vi "Start.vi"(5 "ShowPanel?":bool, 6 "BcQueName":string, 7 "BusIndex":u32, 8 "error in (no error)":errorcluster, 9 "Script":string[](array[string]), 10 "Name":string, 11 "VI Refnum":refnum<vi>) -> (0 "error out":errorcluster, 2 "BC ID":i32, 3 "BCAdmin":refnum<class "BCAdmin.lvclass">)   [LabVIEW 2014, in "BusController.lvlib"]
uses:
  BusController.lvlib
  Admin/BCAdmin.lvclass
  Admin/BCAdmin.lvclass/BCAdmin.ctl
  Admin/Accessors/Write BC ID.vi
  Admin/Accessors/Write BCRegRef.vi
  Admin/Accessors/Write Name.vi
  Admin/Accessors/Write Script.vi
  Admin/Accessors/Write BusIndex.vi
  Admin/Accessors/Write BcQueName.vi
  Admin/Accessors/Write ShowPanel_.vi
  <vilib>/Utility/error.llb/Error Cluster From Error Code.vi
  <vilib>/ErrorRing/Error Ring.xnode
  Admin/Registry/BCReg.lvclass
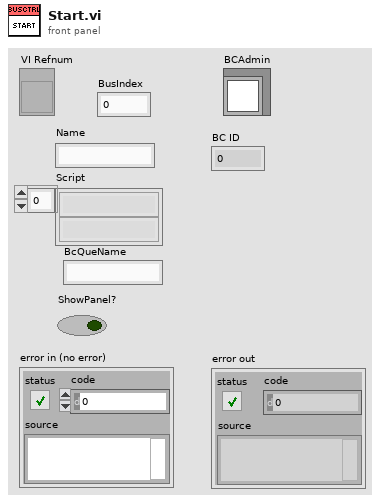
[diagram p1: front panel]
types:
  T1 = enum32{"Bad", "Idle", "Run top level", "Running"}
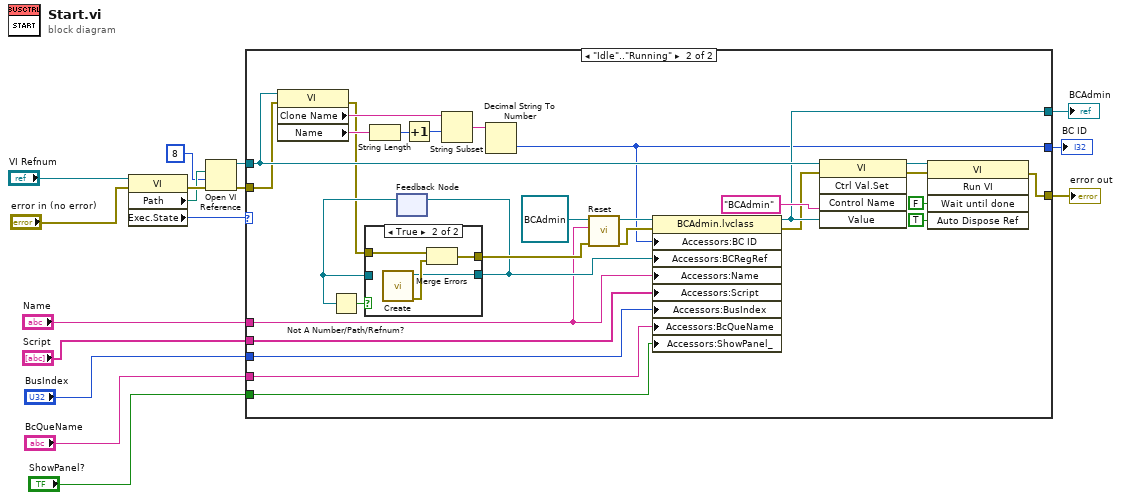
[diagram p0: block diagram]
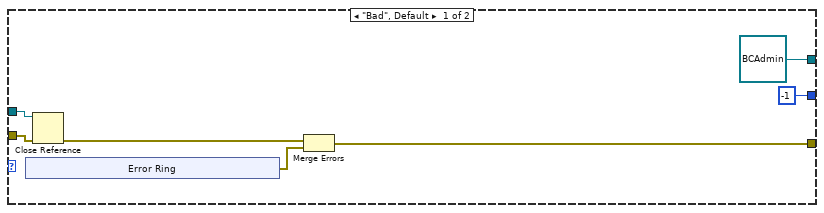
[diagram p2: hidden frame]
diagram:
  n1 = property class="VI"(reference="VI Refnum", error in="error in (no error)") -> (error out=w13:errorcluster, "Path"=w12:path, "Exec.State"=w14:T1)  [unwired: 1 out]
  n2 = Open VI Reference(vi path=w12, options=8, error in (no error)=w13) -> (vi reference=w9:refnum<vi>, error out=w10:errorcluster)  [unwired: 3 in]
  n3 = case shown="\"Idle\"..\"Running\"" w14 {
    tunnel: w10 -> [w22 w33]
    tunnel: w9 -> [w23 w43]
    tunnel: [w19 w37] -> w8
    tunnel: [refnum<class "BCAdmin.lvclass"> refnum ("BCAdmin") w36] -> w7
    tunnel: "Name" -> [_ w44]
    tunnel: [-1 w35] -> w5
    tunnel: "Script" -> [_ w34]
    tunnel: "BusIndex" -> [_ w30]
    tunnel: "BcQueName" -> [_ w29]
    tunnel: "ShowPanel?" -> [_ w28]
    frame "Bad", Default {
      n4 = xnode "Error Ring"() -> ("error out"=w20:errorcluster)
      n5 = Close Reference(reference=w23, error in (no error)=w22) -> (error out=w21:errorcluster)
      n6 = Merge Errors(w21, w20) -> (w19:errorcluster)
    }
    frame "Idle".."Running" {
      n7 = property class="VI"(reference=w43, error in=w33) -> (error out=w32:errorcluster, "Clone Name"=w55:string, "Name"=w52:string)  [unwired: 1 out]
      n8 = String Length(string=w52) -> (length=w53:i32)
      n9 = feedback #1() -> (w50:refnum<data-value>)  [unwired: 1 in]
      n10 = Not A Number/Path/Refnum?(number/path/refnum=w50) -> (NaN/Path/Refnum?=w51:bool)
      n11 = case shown="True" w51 {
        tunnel: [w58 w61] -> w45
        tunnel: [w57 w60] -> w48
        tunnel: w32 -> [w57 w59]
        tunnel: w50 -> [w58 _]
        frame False {
        }
        frame True {
          n12 = call "Create.vi"() -> ("error out"=w62:errorcluster, "BCReg"=w61:refnum<data-value>)  [unwired: 10 in]
          n13 = Merge Errors(w59, w62) -> (w60:errorcluster)
        }
      }
      n14 = feedback-in #1(w45) -> ()
      n15 = Increment(x=w53) -> (x+1=w54:i32)
      n16 = String Subset(string=w55, offset (0)=w54) -> (substring=w56:string)  [unwired: 1 in]
      n17 = Decimal String To Number(string=w56) -> (number=w35:i32)  [unwired: 2 in, 1 out]
      n18 = call "Reset.vi"("error in (no error)"=w48, "Name"=w44, "BCAdmin"=refnum<class "BCAdmin.lvclass"> refnum ("BusController.lvlib:BCAdmin.lvclass")) -> ("error out"=w46:errorcluster, "BCAdmin 2"=w47:refnum<class "BCAdmin.lvclass">)  [unwired: 7 in]
      n19 = property class="BCAdmin.lvclass"(reference=w47, error in=w46, "Accessors:BC ID"=w35, "Accessors:BCRegRef"=w45, "Accessors:Name"=w44, "Accessors:Script"=w34, "Accessors:BusIndex"=w30, "Accessors:BcQueName"=w29, "Accessors:ShowPanel_"=w28) -> (reference out=w36:refnum<class "BCAdmin.lvclass">, error out=w31:errorcluster)
      n20 = invoke class="VI" method="Ctrl Val.Set"(reference=w43, error in=w31, "Control Name"="BCAdmin", "Value"=w36) -> (reference out=w41:refnum<vi>, error out=w40:errorcluster)  [unwired: 1 in, 3 out]
      n21 = invoke class="VI" method="Run VI"(reference=w41, error in=w40, "Wait until done"=FALSE ("Wait Until Done"), "Auto Dispose Ref"=TRUE ("Auto Dispose Reference")) -> (error out=w37:errorcluster)  [unwired: 1 in, 4 out]
    }
  }
  "error out" <- w8
  "BCAdmin" <- w7
  "BC ID" <- w5
